vi "Exclude Conpane Item.vi"(8 "error in (no error)":errorcluster, 9 "Rectangle":T1, 10 "Fully Qualified Array":string[](array[string]), 11 "Control in":refnum<vi>) -> (0 "error out":errorcluster, 2 "Exclude?":bool, 3 "Control out":refnum<vi>)   [LabVIEW 2020, in "Message Maker.lvlib"]
uses:
  Message Maker.lvlib
  <vilib>/Utility/miscctls.llb/LVRectTypeDef.ctl
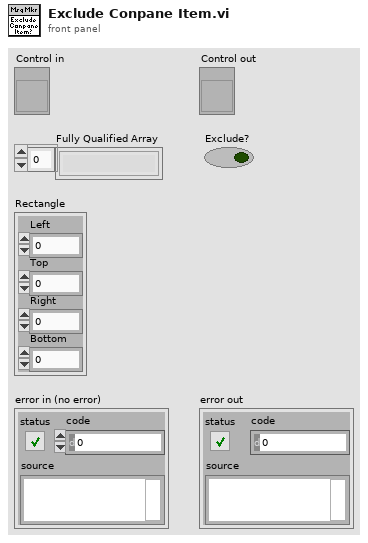
[diagram p1: front panel]
types:
  T1 = typedef "LVRectTypeDef.ctl" = cluster{"Left":i16, "Top":i16, "Right":i16, "Bottom":i16}
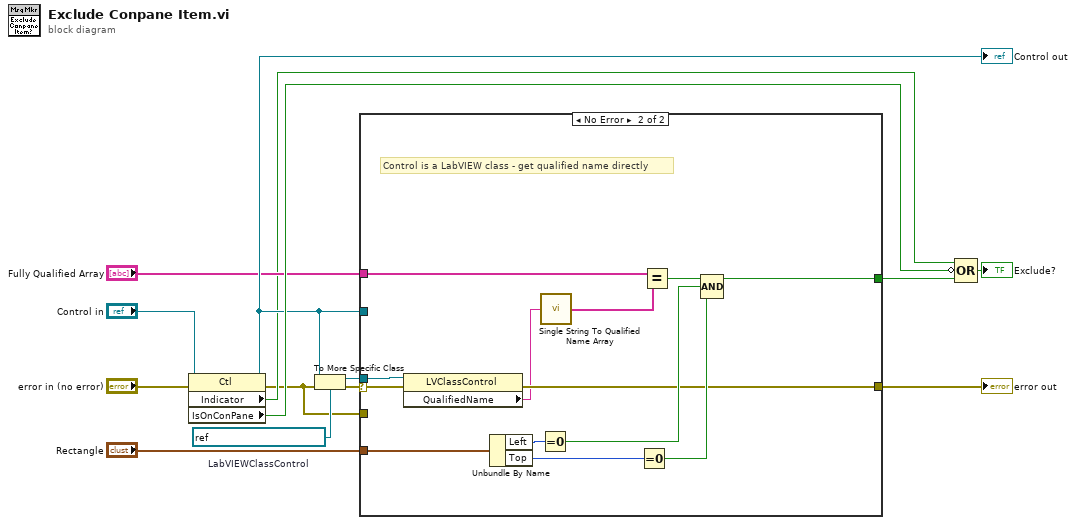
[diagram p0: block diagram]
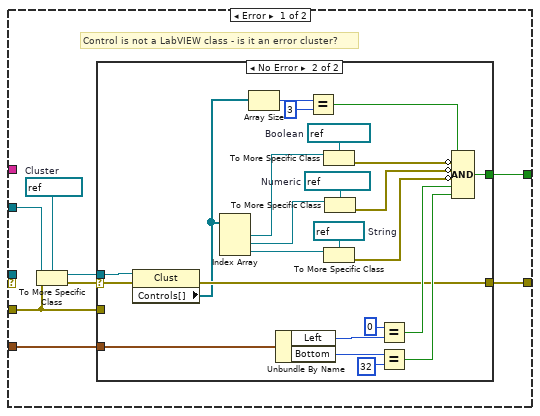
[diagram p2: hidden frame]
diagram:
  w4 = refnum<vi> refnum  # LabVIEWClassControl
  n1 = property class="Ctl"(reference="Control in", error in="error in (no error)") -> (reference out=w12:refnum<vi>, error out=w1:errorcluster, "Indicator"=w6:bool, "IsOnConPane"=w14:bool)
  "Control out" <- w12
  n2 = To More Specific Class(target class=w4, reference=w12, error in=w1) -> (specific class reference=w2:refnum<vi>, error out=w3:errorcluster)
  n3 = case shown="No Error" w3 {
    selector: w3 -> [_ w51]
    tunnel: [w20 w56] -> w7
    tunnel: "Fully Qualified Array" -> [_ w60]
    tunnel: [w21 w50] -> w11
    tunnel: "Rectangle" -> [w22 w57]
    tunnel: w2 -> [_ w52]
    tunnel: w12 -> [w18 _]
    tunnel: w1 -> [w15 _]
    frame Error {
      w19 = refnum<vi> refnum  # Cluster
      # "Control is not a LabVIEW class - is it an error cluster?"
      n4 = To More Specific Class(target class=w19, reference=w18, error in=w15) -> (specific class reference=w16:refnum<vi>, error out=w17:errorcluster)
      n5 = case shown="No Error" w17 {
        selector: w17 -> [_ w34]
        tunnel: [_ w47] -> w20
        tunnel: [w23 w28] -> w21
        tunnel: w22 -> [_ w46]
        tunnel: w16 -> [_ w33]
        tunnel: w15 -> [w23 _]
        frame Error {
        }
        frame No Error {
          w37 = refnum<vi> refnum  # String
          w36 = refnum<vi> refnum  # Numeric
          w35 = refnum<vi> refnum  # Boolean
          n6 = property class="Clust"(reference=w33, error in=w34) -> (error out=w28:errorcluster, "Controls[]"=w27:refnum<vi>[])  [unwired: 1 out]
          n7 = Index Array(array=w27) -> (element #1=w38:refnum<vi>, element #2=w32:refnum<vi>, element #3=w39:refnum<vi>)  [unwired: 3 in]
          n8 = Array Size(array=w27) -> (size(s)=w26:i32)
          n9 = Unbundle By Name(w46) -> ("Left"=w45:i16, "Bottom"=w44:i16)
          n10 = Equal?(x=w26, y=3) -> (x = y?=w24:bool)
          n11 = To More Specific Class(target class=w35, reference=w38) -> (error out=w31:errorcluster)  [unwired: 1 in, 1 out]
          n12 = To More Specific Class(target class=w37, reference=w39) -> (error out=w29:errorcluster)  [unwired: 1 in, 1 out]
          n13 = To More Specific Class(target class=w36, reference=w32) -> (error out=w30:errorcluster)  [unwired: 1 in, 1 out]
          n14 = Equal?(x=i16 0, y=w45) -> (x = y?=w41:bool)
          n15 = Equal?(x=w44, y=i16 32) -> (x = y?=w40:bool)
          n16 = Compound Arithmetic op=AND(w24, invert w31, invert w30, invert w29, w41, w40) -> (w47:bool)
        }
      }
    }
    frame No Error {
      # "Control is a LabVIEW class - get qualified name directly"
      n17 = property class="LVClassControl"(reference=w52, error in=w51) -> (error out=w50:errorcluster, "QualifiedName"=w49:string)  [unwired: 1 out]
      n18 = Unbundle By Name(w57) -> ("Left"=w58:i16, "Top"=w54:i16)
      n19 = Equal To 0?(x=w58) -> (x = 0?=w55:bool)
      n20 = call <vilib>:"Single String To Qualified Name Array.vi"("Fully Qualified String"=w49) -> ("Fully Qualified Array"=w48:string[])
      n21 = Equal To 0?(x=w54) -> (x = 0?=w53:bool)
      n22 = Equal?(x=w60, y=w48) -> (x = y?=w59:bool)
      n23 = Compound Arithmetic op=AND(w59, w55, w53) -> (w56:bool)
    }
  }
  "error out" <- w11
  n24 = Compound Arithmetic op=OR(w6, invert w14, w7) -> (→"Exclude?":bool)
